vi "sv_UFF58 Init Channels.vi"(0 "function refnum":refnum<k20>, 5 "channel name":string, 11 "error in (no error)":errorcluster) -> (4 "dup function refnum":refnum<k20>, 6 "channel refnum":refnum<k20>, 15 "error out":errorcluster)   [LabVIEW 2017, in "SoundVib_UFF58.lvlib"]
doc: "This VI create a <B>channel refnum</B> for the given <B>function refnum</B>"
uses:
  <vilib>/addons/Sound and Vibration/svt_UFF58/SoundVib_UFF58.lvlib
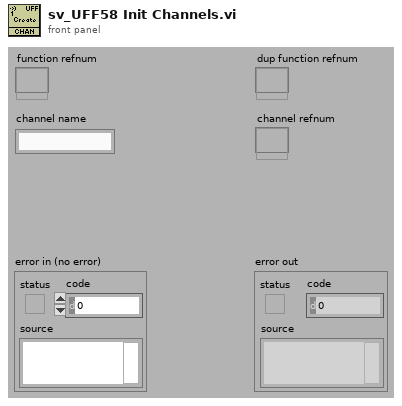
[diagram p1: front panel]
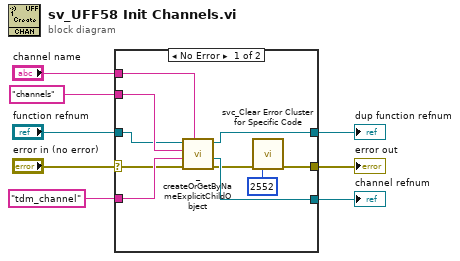
[diagram p0: block diagram]
diagram:
  n1 = case shown="No Error" "error in (no error)" {
    selector: "error in (no error)" -> [w12 w20]
    tunnel: "channels" ("Property name") -> [w18 _]
    tunnel: "tdm_channel" ("Object type") -> [w17 _]
    tunnel: "function refnum" -> [w16 w19]
    tunnel: [w15 w19] -> w5
    tunnel: "channel name" -> [w14 _]
    tunnel: [w13 _] -> w3
    tunnel: [w10 w20] -> w1
    frame No Error {
      n2 = call <vilib>:"_createOrGetByNameExplicitChildObject.vi"("name"=w14, "error in (no error)"=w12, "Object type"=w17, "Property name"=w18, "storage refnum"=w16) -> ("error out"=w11:errorcluster, "new storage refnum"=w13:refnum<k20>, "dup storage refnum"=w15:refnum<k20>)  [unwired: 4 in]
      n3 = call <vilib>:"svc_Clear Error Cluster for Specific Code.vi"("error in (no error)"=w11, "code"=2552 ("warning code")) -> ("error out"=w10:errorcluster)  [unwired: 12 in, 1 out]
    }
    frame Error {
    }
  }
  "error out" <- w1
  "dup function refnum" <- w5
  "channel refnum" <- w3
